vi "Generate Construction Cards.vi"(11 "Path":path) -> (2 "Effect Types":string[](array[string]), 3 "Construction Cards":variant[](array[variant]))   [LabVIEW 2019]
doc: "Array of all cards in game is stored as Variants with key-value pairs. Each card has an Effect (string) and a Value (numeric). Because the images are shared between Effect Types, the images are stored in a separate array."
panel:
  out "size(s)":i32
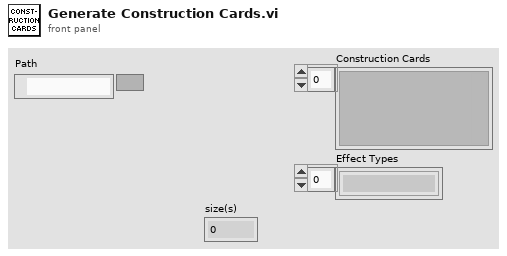
[diagram p1: front panel]
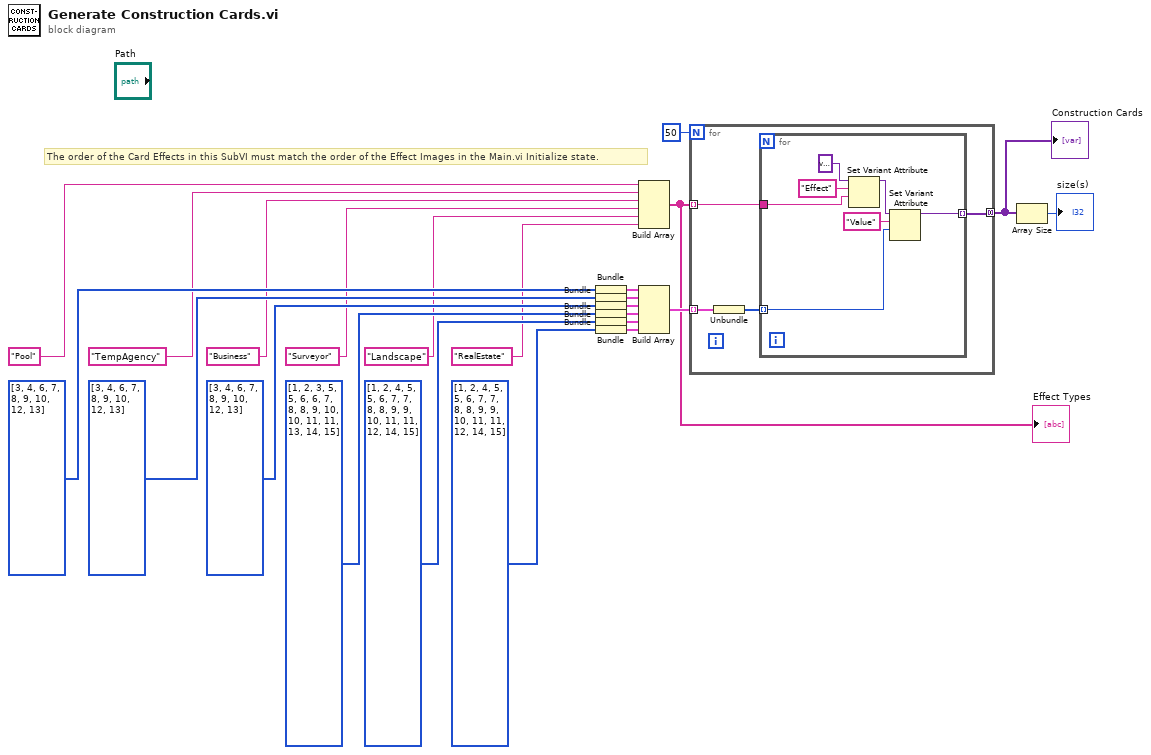
[diagram p0: block diagram]
diagram:
  # "The order of the Card Effects in this SubVI must match the order of the Effect Images in the Main.vi Initialize state."
  n1 = Bundle(i32[] [3, 4, 6, 7, 8, 9, 10, 12, 13]) -> (w8:cluster{i32[]})  [unwired: 1 in]
  n2 = Bundle(i32[] [3, 4, 6, 7, 8, 9, 10, 12, 13]) -> (w9:cluster{i32[]})  [unwired: 1 in]
  n3 = Bundle(i32[] [3, 4, 6, 7, 8, 9, 10, 12, 13]) -> (w10:cluster{i32[]})  [unwired: 1 in]
  n4 = Bundle(i32[] [1, 2, 3, 5, 5, 6, 6, 7, 8, 8, 9, 10, 10, 11, 11, 13, 14, 15]) -> (w11:cluster{i32[]})  [unwired: 1 in]
  n5 = Bundle(i32[] [1, 2, 4, 5, 5, 6, 7, 7, 8, 8, 9, 9, 10, 11, 11, 12, 14, 15]) -> (w12:cluster{i32[]})  [unwired: 1 in]
  n6 = Bundle(i32[] [1, 2, 4, 5, 5, 6, 7, 7, 8, 8, 9, 9, 10, 11, 11, 12, 14, 15]) -> (w13:cluster{i32[]})  [unwired: 1 in]
  n7 = Build Array("Pool", "TempAgency", "Business", "Surveyor", "Landscape", "RealEstate") -> (w1:string[])
  "Effect Types" <- w1
  n8 = Build Array(w8, w9, w10, w11, w12, w13) -> (w22:cluster{i32[]}[])
  n9 = for {
    N: 50 -> [_]
    tunnel: [w27] -> w21 mode=concatenating
    tunnel: w1 -> [w26] mode=indexing
    tunnel: w22 -> [w25] mode=indexing
    n10 = Unbundle(w25) -> (w24:i32[])
    n11 = for {
      tunnel: [w30] -> w27 mode=indexing
      tunnel: w26 -> [w29]
      tunnel: w24 -> [w28] mode=indexing
      n12 = Set Variant Attribute(Variant=variant, name="Effect", value=w29) -> (Variant out=w31:variant)  [unwired: 1 in, 2 out]
      n13 = Set Variant Attribute(Variant=w31, name="Value", value=w28) -> (Variant out=w30:variant)  [unwired: 1 in, 2 out]
    }
  }
  "Construction Cards" <- w21
  n14 = Array Size(array=w21) -> (size(s)=→"size(s)":i32)
